vi "H5Pget_buffer.vi"(6 "error in (no error)":errorcluster, 9 "HDF5 Property Ref":T1) -> (0 "error out":errorcluster, 2 "Buffer Size":u64=1048576, 3 "HDF5 Ref out":T1)   [LabVIEW 2017]
doc: "Reads buffer settings."
uses:
  <vilib>/UPVI/lvhdf5/library.llb/HDF5 Ref.ctl
  <vilib>/UPVI/lvhdf5/hdf5.dll
panel:
  # "LVHDF5 Toolkit\nCopyright (c) 2005-2013 by Jason D. Sommerville\nCopyright (c) 2014 by UPVI, LLC.\n\nThis use and distribution of this file is governed by the terms found in \nLICENSE.txt distributed with this toolkit and installed at\n <user.lib>\\_lvhdf5\\LICENSE.txt"
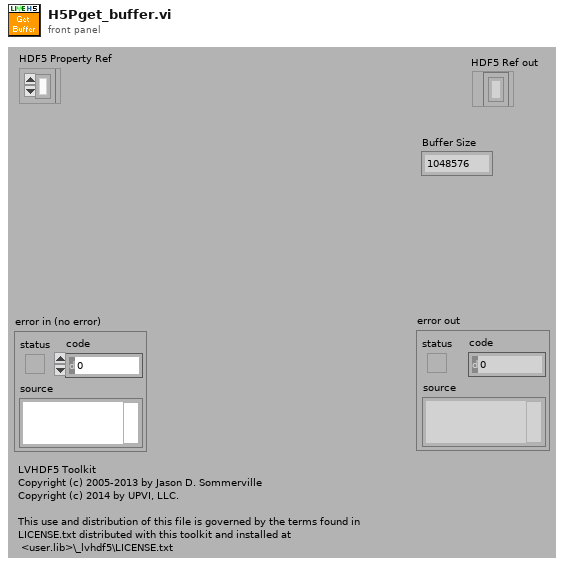
[diagram p1: front panel]
types:
  T1 = typedef "HDF5 Ref.ctl" = refnum<k1>
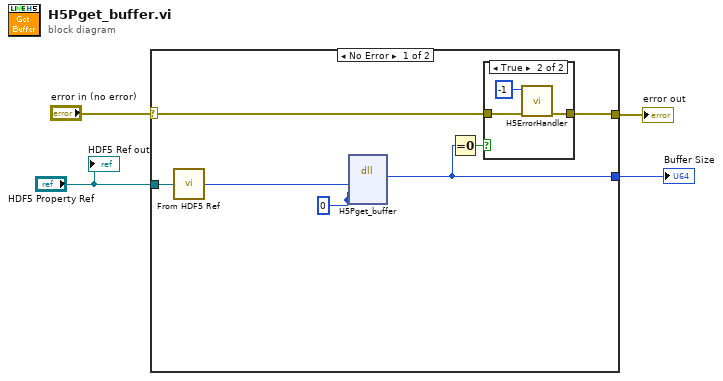
[diagram p0: block diagram]
diagram:
  n1 = case shown="No Error" "error in (no error)" {
    selector: "error in (no error)" -> [w11 w16]
    tunnel: [w10 w16] -> w3
    tunnel: "HDF5 Property Ref" -> [w9 _]
    tunnel: [w6 _] -> w1
    frame No Error {
      w7 = u32 0 ("tconv")
      n2 = call <vilib>:"From HDF5 Ref.vi"("HDF5 Ref"=w9) -> ("I32"=w8:i32)
      n3 = dll-call lib="C:/Program Files/National Instruments/LabVIEW 2017/vi.lib/UPVI/lvhdf5/hdf5.dll" fn="H5Pget_buffer" label="H5Pset_buffer"("plist_id"=w8, "tconv"=w7, "bkg"=w7) -> ("return type"=w6:u64)  [unwired: 6 in, 2 out]
      n4 = Equal To 0?(x=w6) -> (x = 0?=w5:bool)
      n5 = case shown="True" w5 {
        tunnel: w11 -> [w12 w15]
        tunnel: [w12 w14] -> w10
        frame False {
        }
        frame True {
          n6 = call <vilib>:"H5ErrorHandler.vi"("error in (no error)"=w15, "herr_t"=-1) -> ("error out"=w14:errorcluster)  [unwired: 3 in, 4 out]
        }
      }
    }
    frame Error {
    }
  }
  "error out" <- w3
  "Buffer Size" <- w1
  "HDF5 Ref out" <- "HDF5 Property Ref"
